vi "set_ram_data.vi"(11 "ram_data":u8) -> ()   [LabVIEW 2015]
uses:
  <vilib>/rvi/eio/common/nirviEmuTemplateMethod_errors.vi
  <vilib>/eio/EIONode/EIONode.xnode
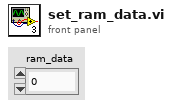
[diagram p1: front panel]
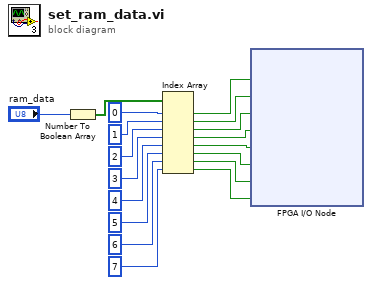
[diagram p0: block diagram]
diagram:
  n1 = Number To Boolean Array(number="ram_data") -> (Boolean array=w1:bool[])
  n2 = Index Array(array=w1, index #1=0 ("index"), index #2=1 ("index"), index #3=2 ("index"), index #4=3 ("index"), index #5=4 ("index"), index #6=5 ("index"), index #7=6 ("index"), index #8=7 ("index")) -> (element #1=w2:bool, element #2=w3:bool, element #3=w4:bool, element #4=w5:bool, element #5=w6:bool, element #6=w7:bool, element #7=w8:bool, element #8=w9:bool)
  n3 = xnode "FPGA I/O Node"("ram_data[0]"=w2, "ram_data[1]"=w3, "ram_data[2]"=w4, "ram_data[3]"=w5, "ram_data[4]"=w6, "ram_data[5]"=w7, "ram_data[6]"=w8, "ram_data[7]"=w9) -> ()  [unwired: 8 in, 8 out]
